vi "CCE RRMA P04 SubVI01.vi"(0 "24-bit pixmap":u32[][](array[numeric]), 1 "umbral superior":u32=127) -> (7 "Array":u32[][](array[numeric]))   [LabVIEW 2020]
doc: "Ceballos Conde Emanuel Rodríguez Ramírez Miguel Ángel 4MV6 Sistemas de visión artificial 2022/1\nEste vi contiene la operacion de binarizacion para el elemento de entrada, obteninendo a la salida 1 si el valor si encuentra dentro del rango dado por el umbral superior e inferior y 0 cuando se encuentra fuera de este rango"
panel:
  # "Ceballos Conde Emanuel\nRodríguez Ramírez Miguel Ángel\n4MV6\nSistemas de visión artificial\n2022/1"
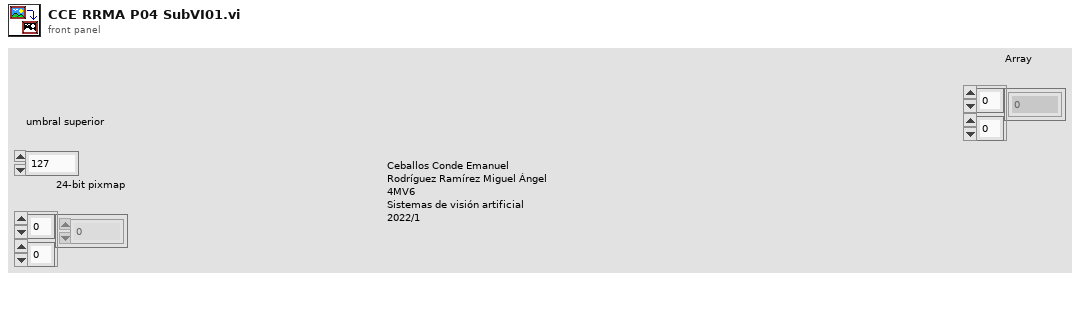
[diagram p1: front panel]
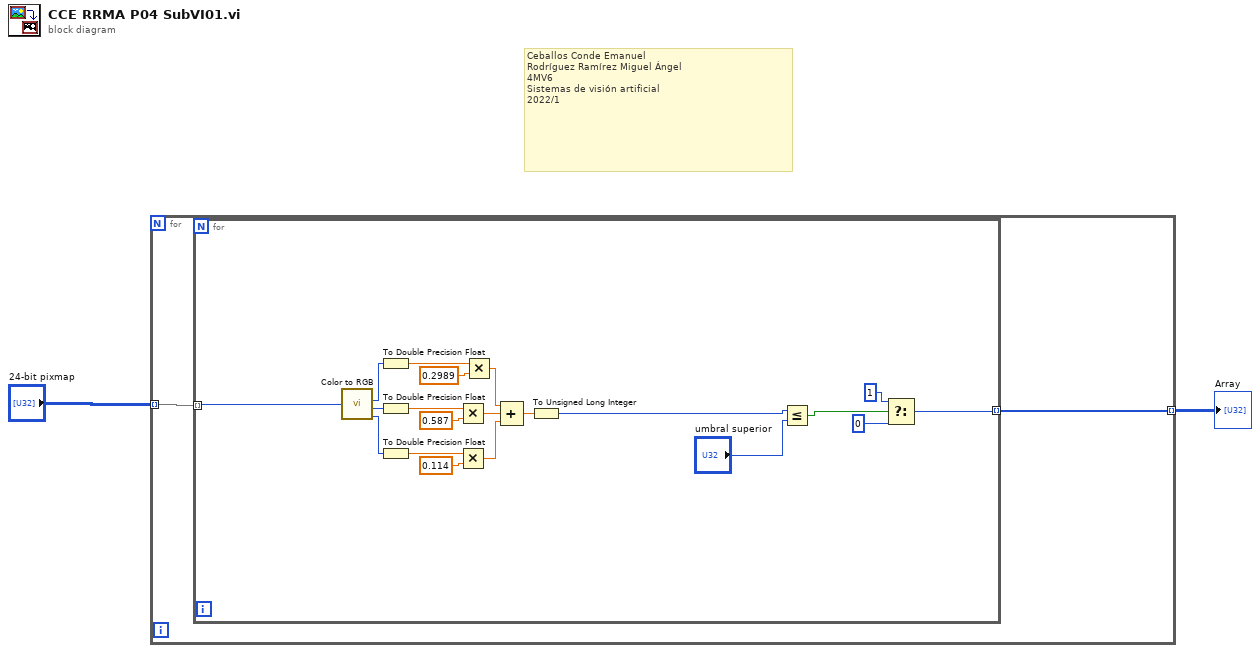
[diagram p0: block diagram]
diagram:
  # "Ceballos Conde Emanuel\nRodríguez Ramírez Miguel Ángel\n4MV6\nSistemas de visión artificial\n2022/1"
  n1 = for {
    tunnel: "24-bit pixmap" -> [w4] mode=indexing
    tunnel: [w3] -> w1 mode=indexing
    n2 = for {
      tunnel: w4 -> [w24] mode=indexing
      tunnel: [w5] -> w3 mode=indexing
      n3 = call <vilib>:"Color to RGB.vi"("Color"=w24) -> ("R"=w23:u8, "G"=w22:u8, "B"=w21:u8)  [unwired: 1 out]
      n4 = To Double Precision Float(number=w23) -> (double precision float=w13:dbl)
      n5 = To Double Precision Float(number=w22) -> (double precision float=w12:dbl)
      n6 = To Double Precision Float(number=w21) -> (double precision float=w11:dbl)
      n7 = Multiply(x=w12, y=0.587) -> (x*y=w16:dbl)
      n8 = Multiply(x=w11, y=0.114) -> (x*y=w15:dbl)
      n9 = Multiply(x=w13, y=0.2989) -> (x*y=w17:dbl)
      n10 = Compound Arithmetic op=ADD(w17, w16, w15) -> (w14:dbl)
      n11 = To Unsigned Long Integer(number=w14) -> (unsigned 32bit integer=w7:u32)
      n12 = Less Or Equal?(x=w7, y="umbral superior") -> (x <= y?=w6:bool)
      n13 = Select(t=u32 1, s=w6, f=u32 0) -> (s? t:f=w5:u32)
    }
  }
  "Array" <- w1
